vi "NGTS_Configure Analog Input Channel.vi"(0 "task in":refnum<k21>, 1 "Channel Address":string, 2 "Channel Name":string, 3 "Units":string, 4 "Custom Scale Name":string, 7 "error in (no error)":errorcluster, 8 "maximum value":dbl=5.0 format="%0.2f", 10 "minimum value":dbl=-5.0 format="%0.2f", 14 "input terminal configuration":i32(ring)=10106 items=["default"=-1, "RSE"=10083, "NRSE"=10078, "Differential"=10106, "Pseudodifferential"=12529]) -> (20 "task out":refnum<k21>, 27 "error out":errorcluster)   [LabVIEW 2018]
doc: "Configures an Analog Input channel as either Voltage\\Amperes\\Basic, or as thermocouple based on finding \"deg\" in the start of the Units input.\n\n2007-11 Mike Ashe"
uses:
  <vilib>/DAQmx/create/channels.llb/DAQmx Create Channel (AI-Voltage-Basic).vi
  <vilib>/DAQmx/create/channels.llb/DAQmx Create Channel (AI-Temperature-Thermocouple).vi
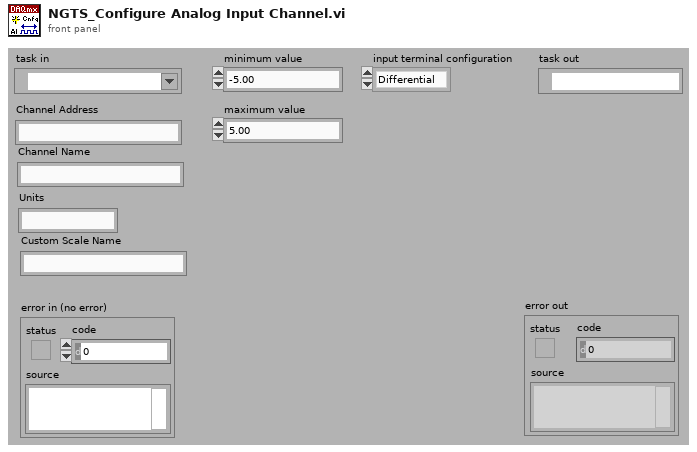
[diagram p1: front panel]
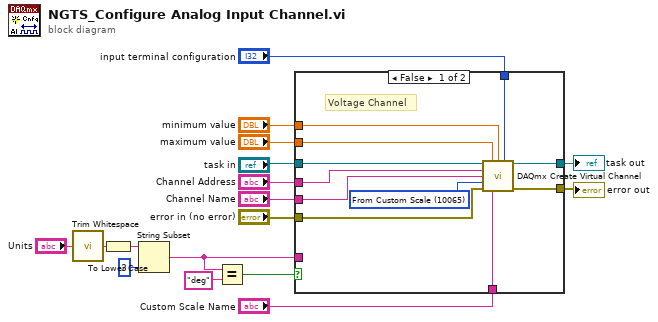
[diagram p0: block diagram]
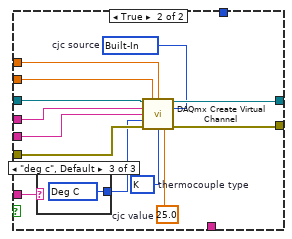
[diagram p2: hidden frame]
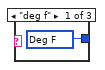
[diagram p3: hidden frame]
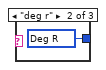
[diagram p4: hidden frame]
diagram:
  n1 = call <vilib>:"Trim Whitespace.vi"("string"="Units") -> ("trimmed string"=w4:string)  [unwired: 1 in]
  n2 = To Lower Case(string=w4) -> (all lower case string=w3:string)
  n3 = String Subset(string=w3, length (rest)=3 ("length (rest)")) -> (substring=w2:string)  [unwired: 1 in]
  n4 = Equal?(x=w2, y="deg") -> (x = y?=w14:bool)
  n5 = case "Temperature Channel" shown="False" w14 {
    tunnel: "task in" -> [w28 w41]
    tunnel: "maximum value" -> [w27 w35]
    tunnel: "minimum value" -> [w26 w36]
    tunnel: "Channel Address" -> [w25 w37]
    tunnel: "Channel Name" -> [w24 w34]
    tunnel: "Custom Scale Name" -> [w22 _]
    tunnel: [w21 w40] -> w7
    tunnel: "error in (no error)" -> [w20 w38]
    tunnel: [w19 w39] -> w5
    tunnel: w2 -> [_ w30]
    tunnel: "input terminal configuration" -> [w18 _]
    frame False {
      w23 = 10065 items=["Volts"=10348, "From Custom Scale"=10065] ("units")
      # "Voltage Channel"
      n6 = call-poly <vilib>:"DAQmx Create Virtual Channel.vi"("task in"=w28, "maximum value"=w27, "minimum value"=w26, "input terminal configuration"=w18, "physical channels"=w25, "name to assign"=w24, "units"=w23, "error in"=w20, "custom scale name"=w22) -> ("task out"=w21:refnum<k21>, "error out"=w19:errorcluster)  [unwired: 5 in]
    }
    frame True {
      w32 = 25.0  # cjc value
      w31 = 10200 items=["Built-In"=10200, "Constant Value"=10116, "Channel"=10113]  # cjc source
      w33 = 10073 items=["J"=10072, "K"=10073, "N"=10077, "R"=10082, "S"=10085, "T"=10086, "B"=10047, "E"=10055]  # thermocouple type
      n7 = case shown="\"deg c\", Default" w30 {
        tunnel: [w42 w43 w44] -> w29
        frame "deg f" {
          w42 = 10144 items=["Deg C"=10143, "Deg F"=10144, "Kelvins"=10325, "Deg R"=10145, "From Custom Scale"=10065] ("units")
        }
        frame "deg r" {
          w43 = 10145 items=["Deg C"=10143, "Deg F"=10144, "Kelvins"=10325, "Deg R"=10145, "From Custom Scale"=10065] ("units")
        }
        frame "deg c", Default {
          w44 = 10143 items=["Deg C"=10143, "Deg F"=10144, "Kelvins"=10325, "Deg R"=10145, "From Custom Scale"=10065] ("units")
        }
      }
      n8 = call-poly <vilib>:"DAQmx Create Virtual Channel.vi"("task in"=w41, "maximum value"=w35, "minimum value"=w36, "physical channels"=w37, "cjc source"=w31, "name to assign"=w34, "units"=w29, "error in"=w38, "thermocouple type"=w33, "cjc value"=w32) -> ("task out"=w40:refnum<k21>, "error out"=w39:errorcluster)  [unwired: 4 in]
    }
  }
  "error out" <- w5
  "task out" <- w7
